vi "TRITON_LOOP_MODE_COMMAND.vi"(1 "Heater Control Mode":enum16{"Open Loop", "Closed Loop"}(ring)=enum."Closed Loop", 2 "Temperature Control Channel":i32=5) -> (0 "Command String":string)   [LabVIEW 2009]
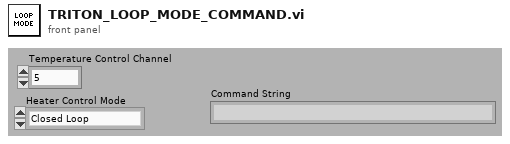
[diagram p1: front panel]
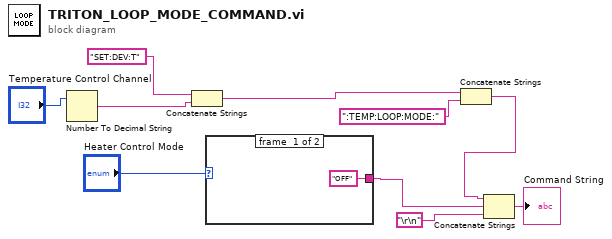
[diagram p0: block diagram]
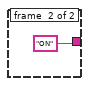
[diagram p2: hidden frame]
diagram:
  n1 = Number To Decimal String(number="Temperature Control Channel") -> (decimal integer string=w5:string)  [unwired: 1 in]
  n2 = Concatenate Strings("SET:DEV:T", w5) -> (w3:string)
  n3 = case shown="\"Closed Loop\"" "Heater Control Mode" {
    tunnel: ["OFF" "ON"] -> w8
    frame #0 {
    }
    frame #1 {
    }
  }
  n4 = Concatenate Strings(w3, ":TEMP:LOOP:MODE:") -> (w2:string)
  n5 = Concatenate Strings(w2, w8, "\r\n") -> (→"Command String":string)
